vi "Gaussian Peak Fit Coefficients.vi"(0 "Y":dbl[](array[numeric]), 1 "initial guess":T1={"initial amplitude"=nan, "initial center"=nan, "initial standard deviation"=nan}, 5 "X":dbl[](array[numeric]), 7 "Weight":dbl[](array[numeric]), 9 "tolerance":dbl=0.0001 format="%#_3g", 11 "method":T2 items=["Least Square", "Least Absolute Residual", "Bisquare"]) -> (4 "amplitude":dbl, 6 "center":dbl, 8 "standard deviation":dbl, 15 "error":i32)   [LabVIEW 2014, in "NI_AALPro.lvlib"]
doc: "Returns the <B>amplitude</B>, <B>center</B>, and <B>standard deviation</B> of the Gaussian fit for a data set (<B>X</B>, <B>Y</B>)."
uses:
  NI_AALPro.lvlib
  Curve Fitting Criteria.ctl
panel:
  # "Gaussian Peak Fit Coefficients"
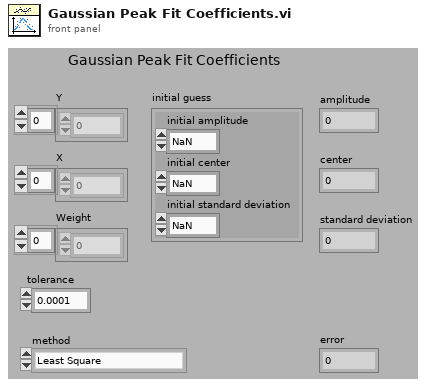
[diagram p1: front panel]
types:
  T1 = cluster{"initial amplitude":dbl, "initial center":dbl, "initial standard deviation":dbl}
  T2 = typedef "NI_AALPro.lvlib/Curve Fitting Criteria.ctl" = u16
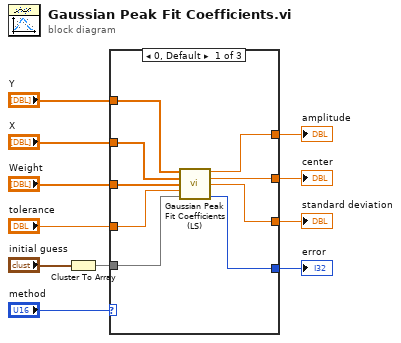
[diagram p0: block diagram]
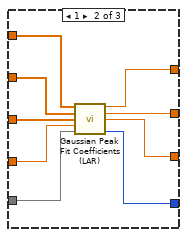
[diagram p2: hidden frame]
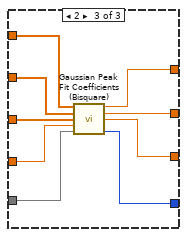
[diagram p3: hidden frame]
diagram:
  n1 = Cluster To Array(cluster="initial guess") -> (array=w1:dbl[])
  n2 = case shown="0, Default" "method" {
    tunnel: "Y" -> [w20 w29 w38]
    tunnel: "X" -> [w19 w28 w37]
    tunnel: "Weight" -> [w18 w27 w36]
    tunnel: "tolerance" -> [w17 w26 w35]
    tunnel: w1 -> [w16 w25 w34]
    tunnel: [w15 w24 w33] -> w6
    tunnel: [w14 w23 w32] -> w5
    tunnel: [w13 w22 w31] -> w4
    tunnel: [w12 w21 w30] -> w3
    frame 0, Default {
      n3 = call "Gaussian Peak Fit Coefficients (LS).vi"("Y"=w20, "X"=w19, "Weight"=w18, "tolerance"=w17, "Initial Coefficients"=w16) -> ("amplitude"=w15:dbl, "center"=w14:dbl, "width"=w13:dbl, "error"=w12:i32)  [unwired: 7 out]
    }
    frame 1 {
      n4 = call "Gaussian Peak Fit Coefficients (LAR).vi"("Y"=w29, "X"=w28, "Weight"=w27, "tolerance"=w26, "Initial Coefficients"=w25) -> ("amplitude"=w24:dbl, "center"=w23:dbl, "width"=w22:dbl, "error"=w21:i32)  [unwired: 7 out]
    }
    frame 2 {
      n5 = call "Gaussian Peak Fit Coefficients (Bisquare).vi"("Y"=w38, "X"=w37, "Weight"=w36, "tolerance"=w35, "Initial Coefficients"=w34) -> ("amplitude"=w33:dbl, "center"=w32:dbl, "width"=w31:dbl, "error"=w30:i32)  [unwired: 7 out]
    }
  }
  "amplitude" <- w6
  "center" <- w5
  "standard deviation" <- w4
  "error" <- w3
